vi "fix default.vi"(10 "input values":dbl[](array[numeric])) -> (3 "fix default":bool)   [LabVIEW 2014]
uses:
  DB_Global_4_kart-Test.vi
panel:
  in  "Kelvin F/P Array":dbl[][](array[numeric])
  in  "1R F/P Array":dbl[][](array[numeric])
  in  "10R F/P Array":dbl[][](array[numeric])
  in  "Wagner F/P Array":dbl[][](array[numeric])
  in  "index r":dbl
  in  "AD F/P Array":dbl[][](array[numeric])
  in  "GPIB In":refnum<visa-resource-name>="GPIB0::8::INSTR"
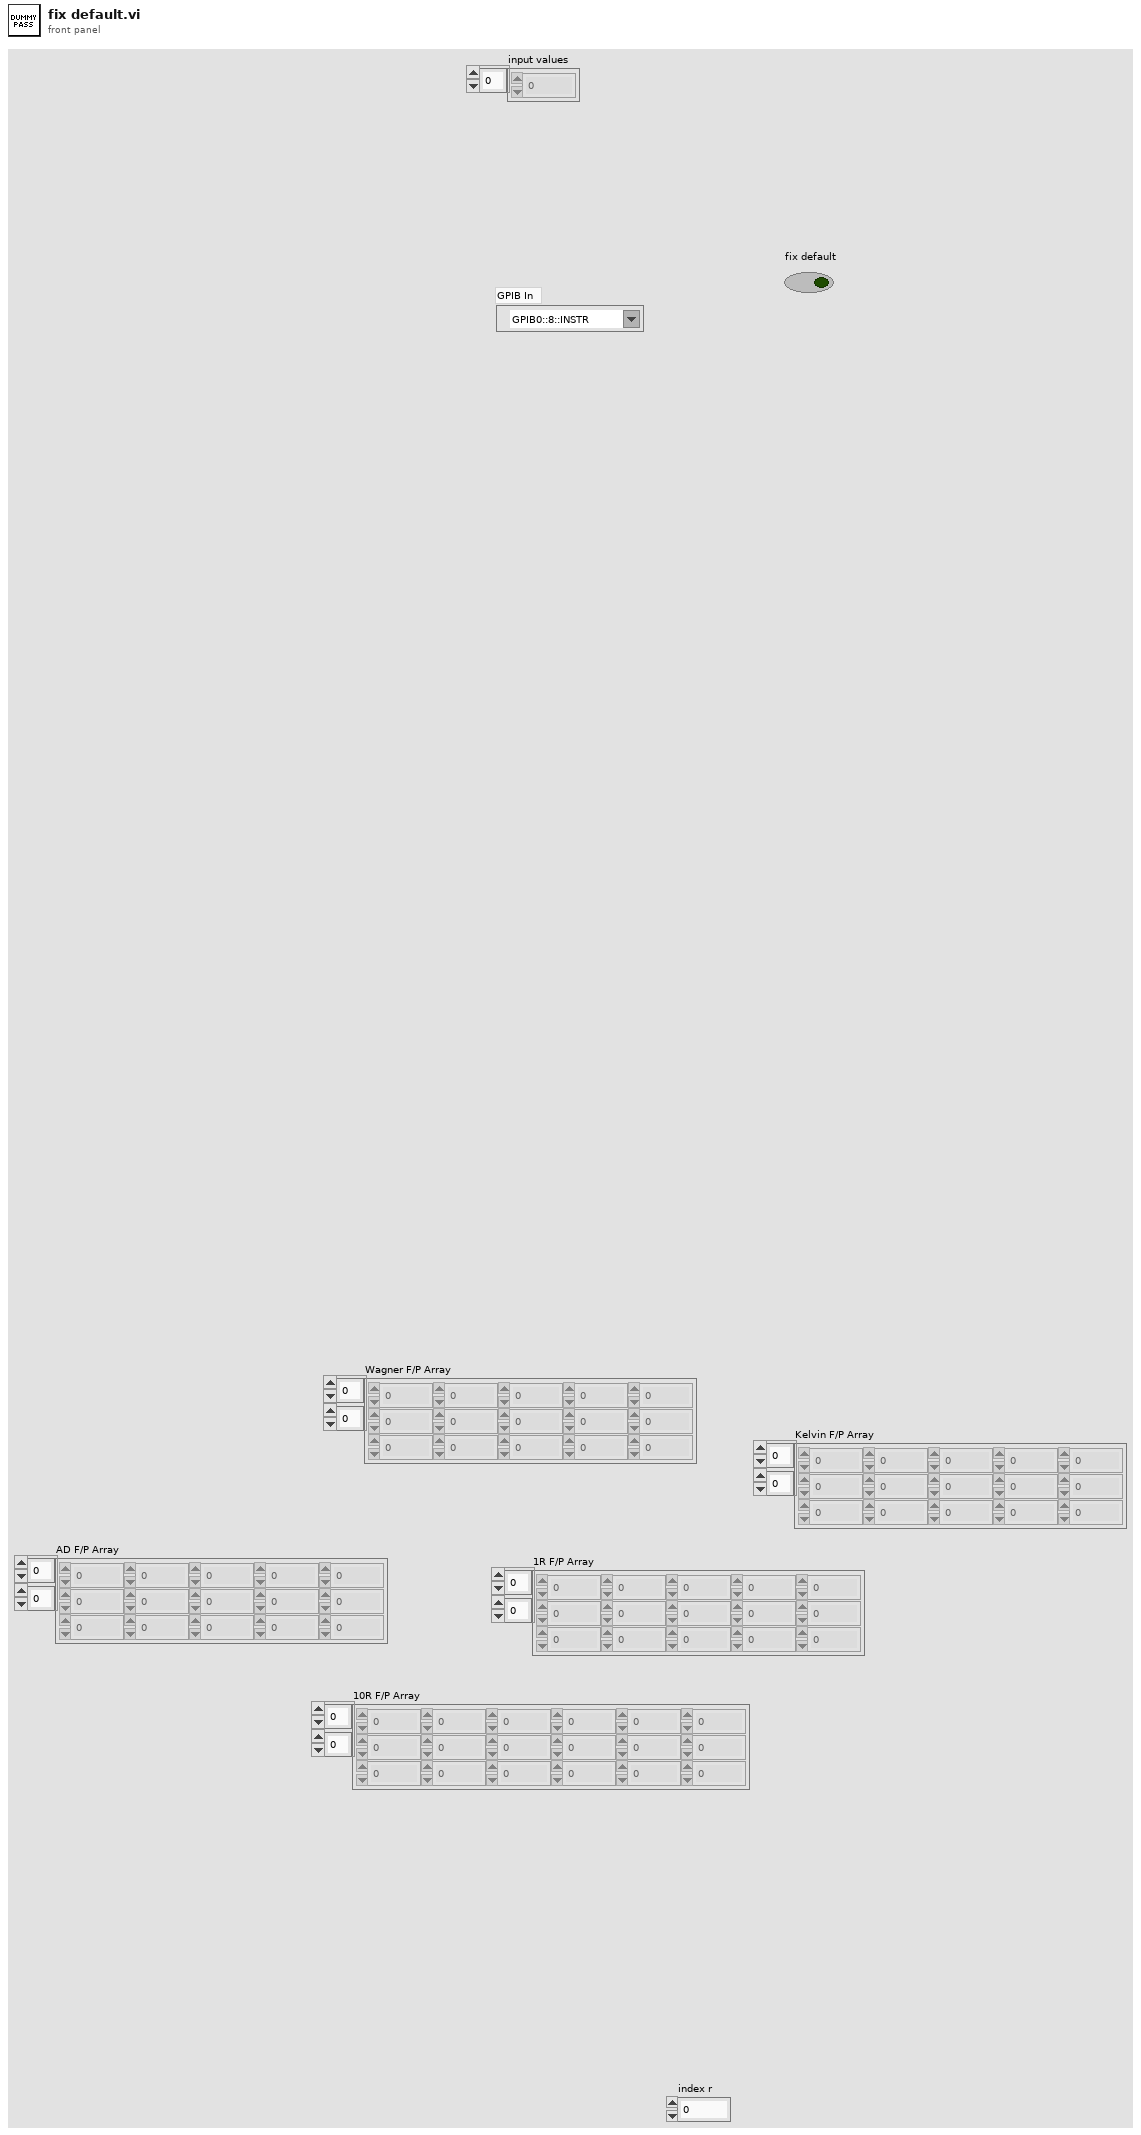
[diagram p1: front panel]
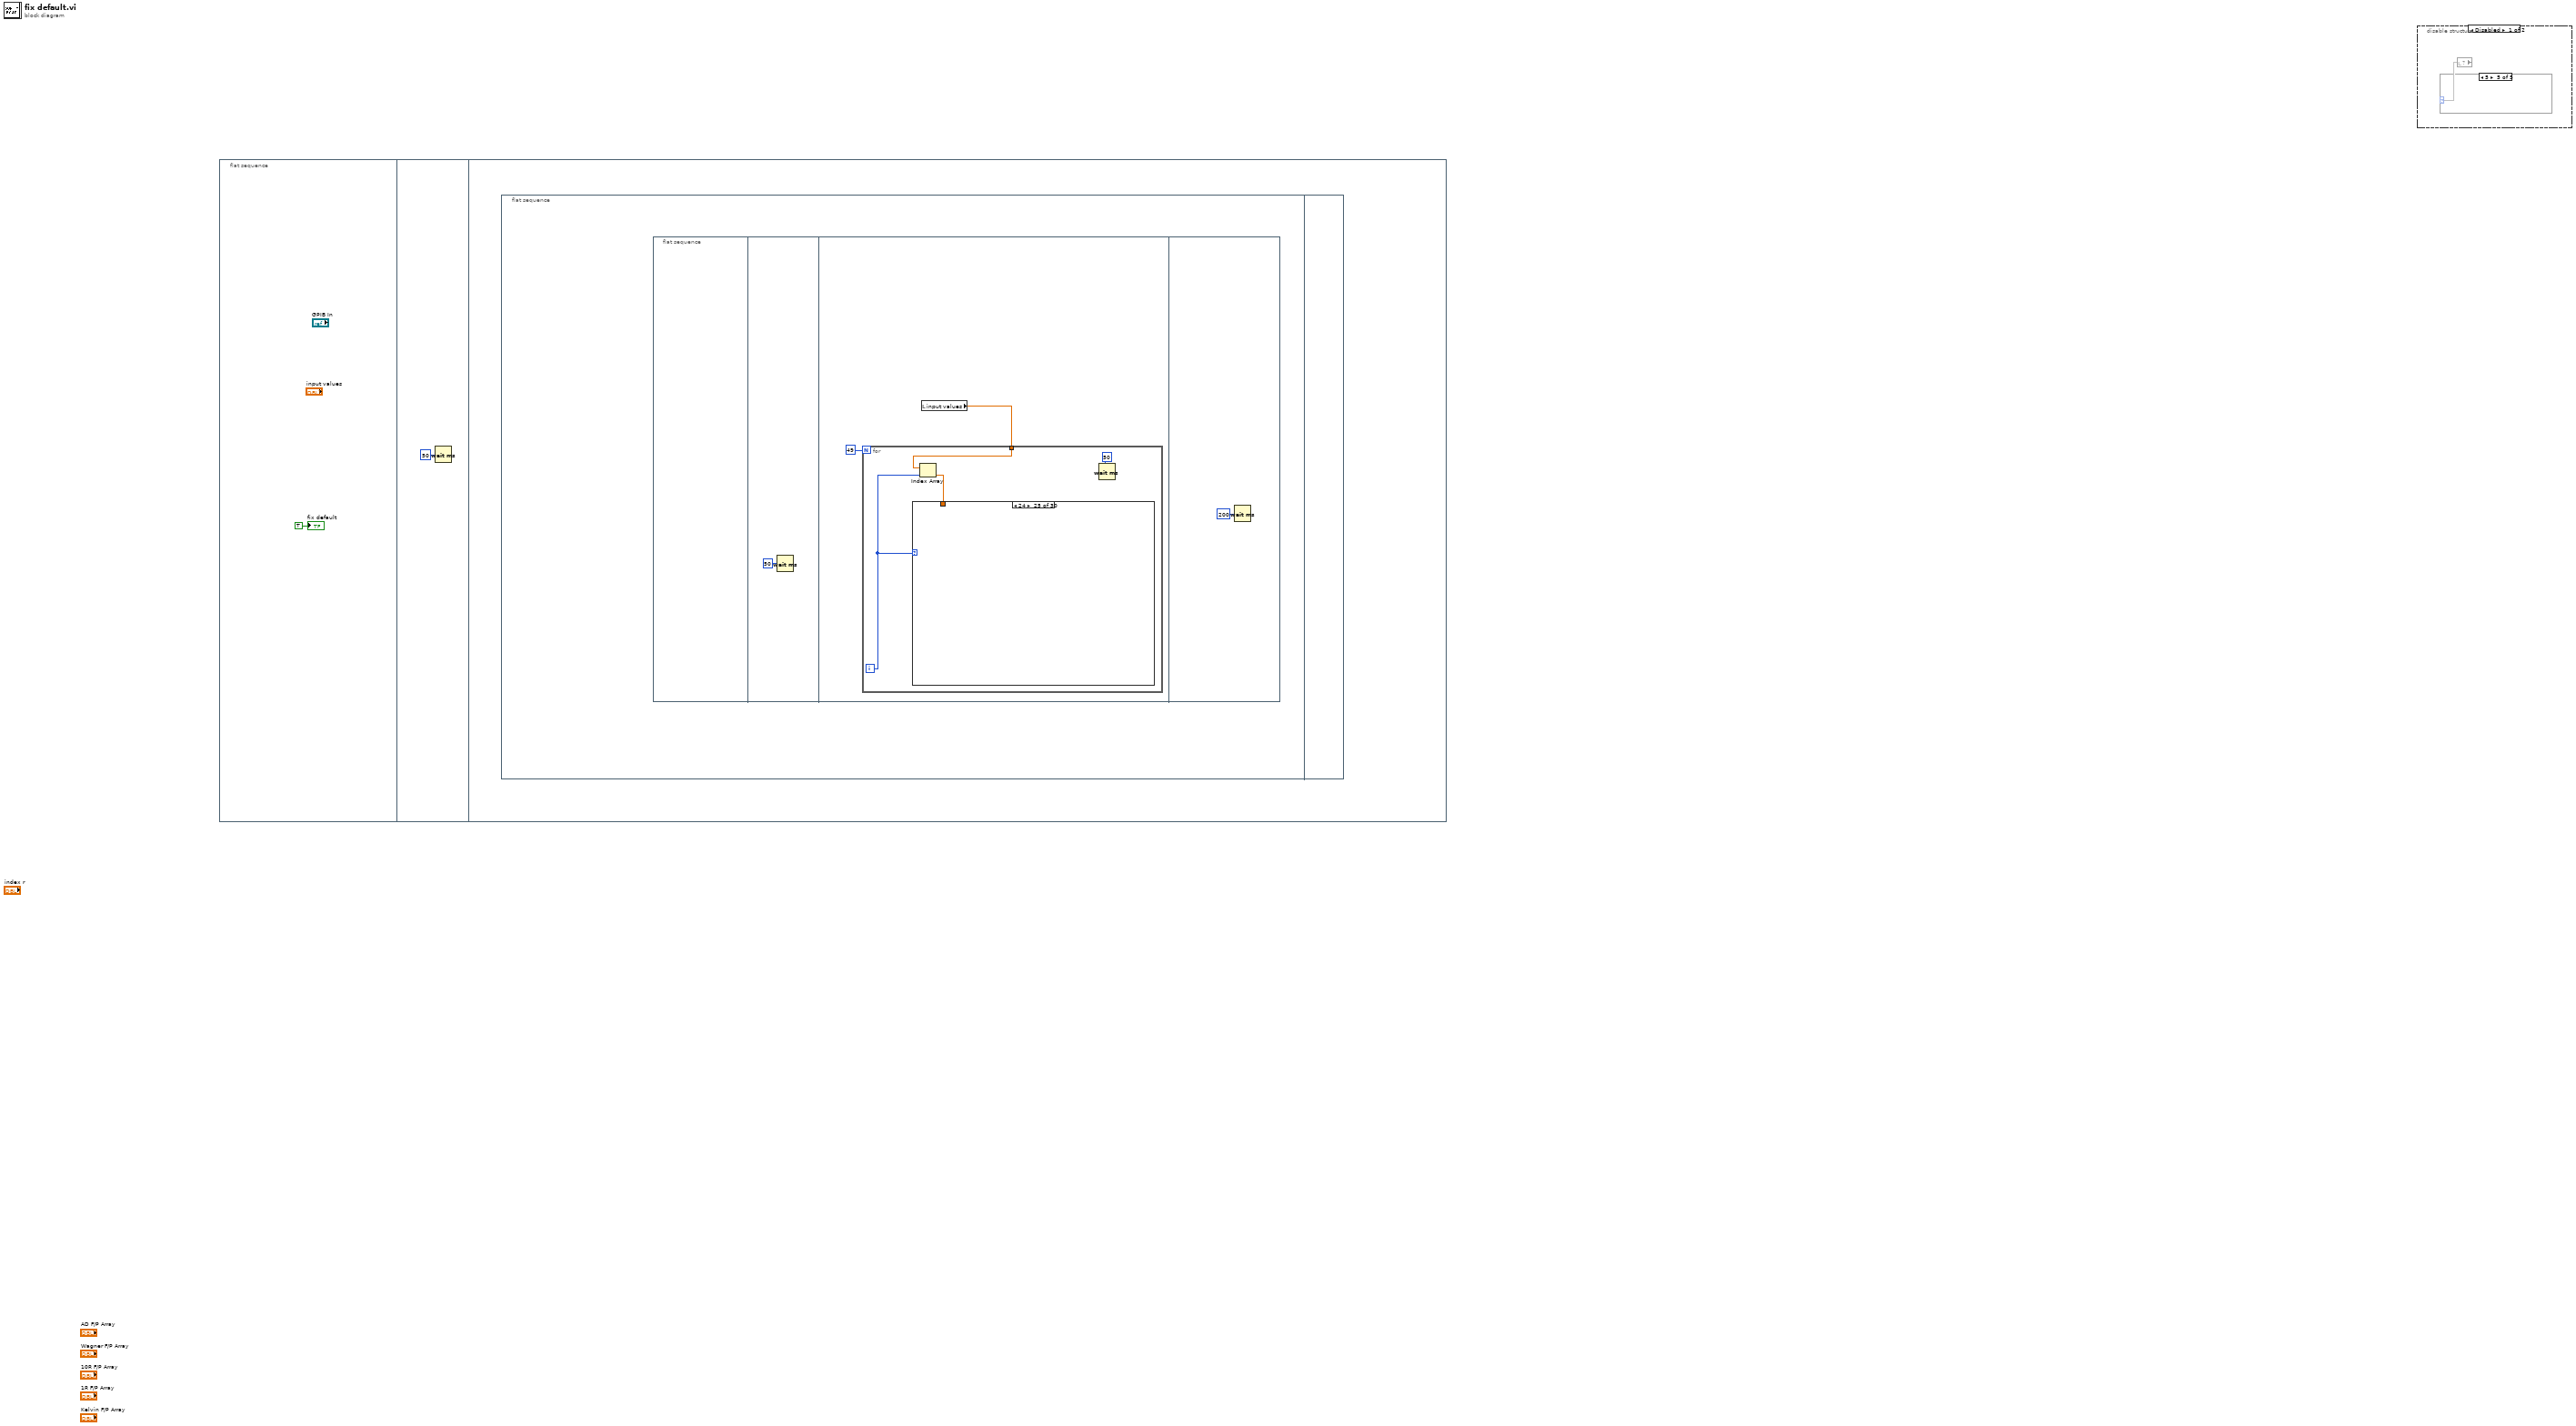
[diagram p0: block diagram]
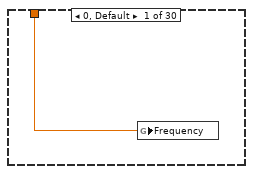
[diagram p2: hidden frame]
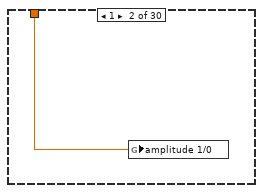
[diagram p3: hidden frame]
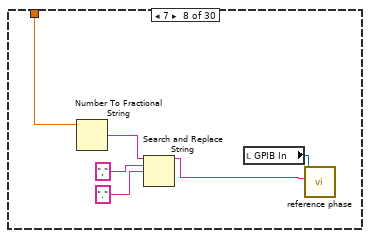
[diagram p9: hidden frame]
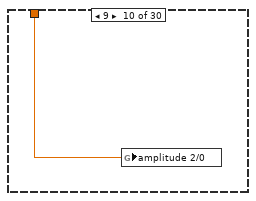
[diagram p11: hidden frame]
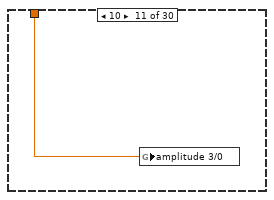
[diagram p12: hidden frame]
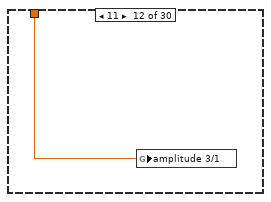
[diagram p13: hidden frame]
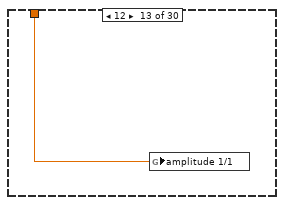
[diagram p14: hidden frame]
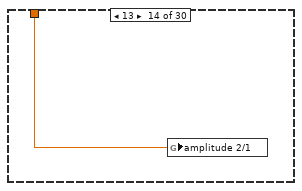
[diagram p15: hidden frame]
diagram:
  n1 = flat-sequence {
    frame #0 {
      "fix default" <- TRUE ("fix default")
    }
    frame #1 {
      n2 = Wait (ms)(milliseconds to wait=u32 50) -> ()  [unwired: 1 out]
    }
    frame #2 {
      n3 = flat-sequence {
        frame #0 {
          n4 = flat-sequence {
            frame #0 {
            }
            frame #1 {
              n5 = Wait (ms)(milliseconds to wait=u32 50) -> ()  [unwired: 1 out]
            }
            frame #2 {
              n6 = local read "input values"() -> (w4:dbl[])
              n7 = for {
                N: 49 -> [_]
                tunnel: w4 -> [w8]
                i -> [w6]
                n8 = Index Array(array=w8, index=w6) -> (element=w7:dbl)
                n9 = case shown="24" w6 {
                  tunnel: w7 -> [w10 w11 _ _ _ _ _ w12 _ w18 w19 w20 w21 w22 _ _ _ _ _ w23 w24 w25 w26 w27 _ _ _ _ _ _]
                  frame 0, Default {
                    n10 = global write "DB_Global_4_kart-Test.vi" "Frequency"(w10) -> ()
                  }
                  frame 1 {
                    n11 = global write "DB_Global_4_kart-Test.vi" "amplitude 1/0"(w11) -> ()
                  }
                  frame 2 {
                  }
                  frame 3 {
                  }
                  frame 4 {
                  }
                  frame 5 {
                  }
                  frame 6 {
                  }
                  frame 7 {
                    n12 = Number To Fractional String(number=w12) -> (F-format string=w15:string)  [unwired: 3 in]
                    n13 = Search and Replace String(input string=w15, search string=",", replace string="." ("replace string (\"\")")) -> (result string=w14:string)  [unwired: 5 in, 3 out]
                    n14 = local read "GPIB In"() -> (w13:refnum<visa-resource-name>)
                    n15 = call "reference phase.vi"("Reference Phase (0.000 degrees)"=w14, "VISA resource name"=w13) -> ()  [unwired: 8 in, 2 out]
                  }
                  frame 8 {
                  }
                  frame 9 {
                    n16 = global write "DB_Global_4_kart-Test.vi" "amplitude 2/0"(w18) -> ()
                  }
                  frame 10 {
                    n17 = global write "DB_Global_4_kart-Test.vi" "amplitude 3/0"(w19) -> ()
                  }
                  frame 11 {
                    n18 = global write "DB_Global_4_kart-Test.vi" "amplitude 3/1"(w20) -> ()
                  }
                  frame 12 {
                    n19 = global write "DB_Global_4_kart-Test.vi" "amplitude 1/1"(w21) -> ()
                  }
                  frame 13 {
                    n20 = global write "DB_Global_4_kart-Test.vi" "amplitude 2/1"(w22) -> ()
                  }
                  frame 14 {
                  }
                  frame 15 {
                  }
                  frame 16 {
                  }
                  frame 17 {
                  }
                  frame 18 {
                  }
                  frame 19 {
                    n21 = global write "DB_Global_4_kart-Test.vi" "phase 2/ 0"(w23) -> ()
                  }
                  frame 20 {
                    n22 = global write "DB_Global_4_kart-Test.vi" "phase 3/0"(w24) -> ()
                  }
                  frame 21 {
                    n23 = global write "DB_Global_4_kart-Test.vi" "phase 3/1"(w25) -> ()
                  }
                  frame 22 {
                    n24 = global write "DB_Global_4_kart-Test.vi" "phase 1/1"(w26) -> ()
                  }
                  frame 23 {
                    n25 = global write "DB_Global_4_kart-Test.vi" "phase 2/1"(w27) -> ()
                  }
                  frame 24 {
                  }
                  frame 25 {
                  }
                  frame 26 {
                  }
                  frame 27 {
                  }
                  frame 28 {
                  }
                  frame 29 {
                  }
                }
                n26 = Wait (ms)(milliseconds to wait=u32 50) -> ()  [unwired: 1 out]
              }
            }
            frame #3 {
              n27 = Wait (ms)(milliseconds to wait=u32 200) -> ()  [unwired: 1 out]
            }
          }
        }
        frame #1 {
        }
      }
    }
  }
  n28 = disable-structure shown="Disabled" {
    frame Disabled {
      n29 = local read item#-1() -> (w29)
      n30 = case shown="5" w29 {
        frame 1 {
        }
        frame 2 {
        }
        frame 3 {
        }
        frame 4, Default {
        }
        frame 5 {
        }
      }
    }
    frame Enabled {
    }
  }
